vi "Stop.vi"(0 "object in":refnum<class "EmergencyController.lvclass">, 2 "Emergancy":bool, 5 "error in (no error)":errorcluster) -> (14 "object out":refnum<class "EmergencyController.lvclass">, 16 "Time(ms)":u32, 19 "error out":errorcluster)   [LabVIEW 2014, in "EmergencyController.lvclass"]
uses:
  EmergencyController.lvclass
  EmergencyController.lvclass/EmergencyController.ctl
  IEmergencyStop_class/IEmergencyStop.lvclass
  Logger_class/Logger.lvclass
  TowerLight_class/TowerLight.lvclass
  ConveyorBelt_class/ConveyorBelt.lvclass
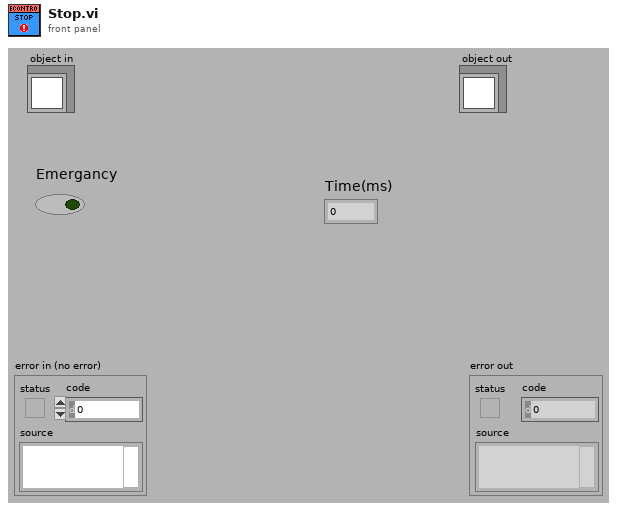
[diagram p1: front panel]
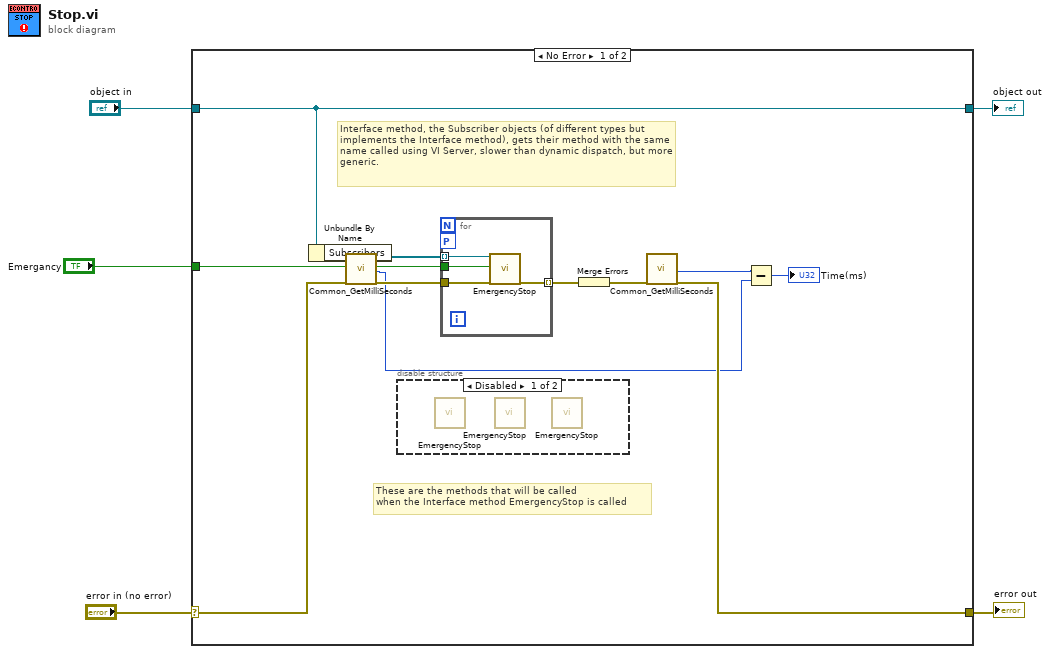
[diagram p0: block diagram]
diagram:
  n1 = case shown="No Error" "error in (no error)" {
    selector: "error in (no error)" -> [w14 w22]
    tunnel: [w9 w22] -> w4
    tunnel: [w16 w21] -> w2
    tunnel: "object in" -> [w16 w21]
    tunnel: "Emergancy" -> [w11 _]
    frame No Error {
      # "These are the methods that will be called\nwhen the Interface method EmergencyStop is called"
      # "Interface method, the Subscriber objects (of different types but implements the Interface method), gets their method with the same name called using VI Server, slower than dynamic dispatch, but more generic."
      n2 = Unbundle By Name(w16) -> ("Subscribers"=w15:refnum<class>[])
      n3 = call "Common_GetMilliSeconds.vi"("error in (no error)"=w14) -> ("msValue"=w7:u32, "error out"=w10:errorcluster)  [unwired: 17 in]
      n4 = disable-structure shown="Disabled" {
        frame Disabled {
          n5 = call-dynamic "EmergencyStop.vi"() -> ()  [unwired: 18 in, 2 out]
          n6 = call-dynamic "EmergencyStop.vi"() -> ()  [unwired: 18 in, 2 out]
          n7 = call-dynamic "EmergencyStop.vi"() -> ()  [unwired: 18 in, 2 out]
        }
        frame Enabled {
        }
      }
      n8 = for {
        tunnel: w15 -> [w20] mode=indexing
        tunnel: w10 -> [w19]
        tunnel: [w18] -> w13 mode=indexing
        tunnel: w11 -> [w17]
        workers-P: _ -> [_]
        n9 = call "EmergencyStop.vi"("Interface In"=w20, "Emergency"=w17, "error in (no error)"=w19) -> ("error out"=w18:errorcluster)  [unwired: 15 in, 1 out]
      }
      n10 = Merge Errors(w13) -> (w12:errorcluster)
      n11 = call "Common_GetMilliSeconds.vi"("error in (no error)"=w12) -> ("msValue"=w8:u32, "error out"=w9:errorcluster)  [unwired: 17 in]
      n12 = Subtract(x=w8, y=w7) -> (x-y=→"Time(ms)":u32)
    }
    frame Error {
    }
  }
  "error out" <- w4
  "object out" <- w2
